vi "Read Relation.vi"(11 "Teller in":refnum<class "Teller.lvclass">) -> (2 "Relation":T1)   [LabVIEW 2025, in "jettl.lvlib" / "Teller.lvlib" / "Teller.lvclass"]
uses:
  Teller.lvclass
  Relation.ctl
  jettl.lvlib
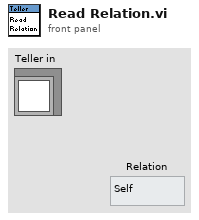
[diagram p1: front panel]
types:
  T1 = typedef "jettl.lvlib/Relation.ctl" = enum16{"Self", "Parent", "Child"}
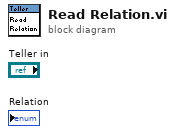
[diagram p0: block diagram]
diagram:
